vi "Verify position.vi"(8 "error in (no error)":errorcluster, 9 "Tolerance (um)":sgl=0.4, 10 "XYZ Position Input":T2={"Speed"=0, "Z Limit (um+/-)"=0.0, "Axes"="Z", "XYZ Coordinates"={"X"=0.0, "Y"=0.0, "Z"=0.0}} {"XYZ Coordinates"."Z" format="Z= %#_g"; "XYZ Coordinates"."Y" format="Y= %#_g"; "XYZ Coordinates"."X" format="X= %#_g"; "Z Limit (um+/-)" format="Z Limit = %.0f"; "Speed" format="Speed= %.0f"}, 11 "Scientifica XYZ Gen1 in":refnum<class "Scientifica XYZ Gen1.lvclass">) -> (0 "error out":errorcluster, 1 "XYZ Coordinates":T1 {"Z" format="Z= %#_g"; "Y" format="Y= %#_g"; "X" format="X= %#_g"}, 2 "Position reached":bool, 3 "Scientifica XYZ Gen1 out":refnum<class "Scientifica XYZ Gen1.lvclass">)   [LabVIEW 2020, in "TranslationStageClassStructure.lvlib" / "Scientifica XYZ Gen1.lvclass"]
uses:
  Scientifica XYZ Gen1.lvclass
  XYZ Stage Control/typedefs/XYZ_position_input.ctl
  XYZ Stage Control/typedefs/XYZ axes.ctl
  Typedefs/XYZ_coordinates.ctl
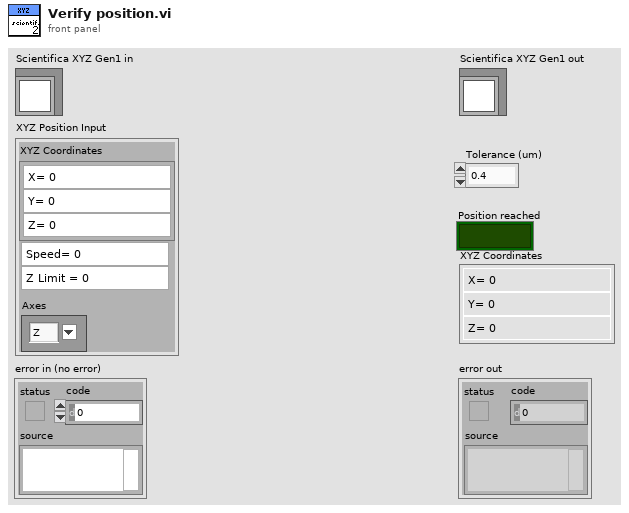
[diagram p1: front panel]
types:
  T1 = typedef "XYZ_coordinates.ctl" = cluster{"X":sgl, "Y":sgl, "Z":sgl}
  T2 = typedef "XYZ_position_input.ctl" = cluster{"Speed":i32, "Z Limit (um+/-)":sgl, "Axes":T3, "XYZ Coordinates":T1}
  T3 = typedef "XYZ axes.ctl" = string
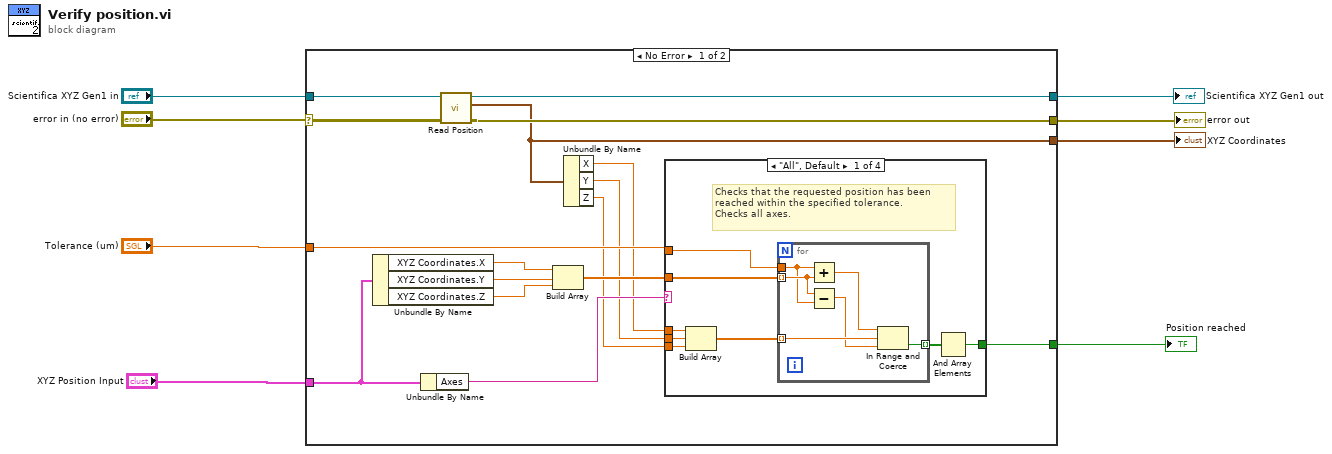
[diagram p0: block diagram]
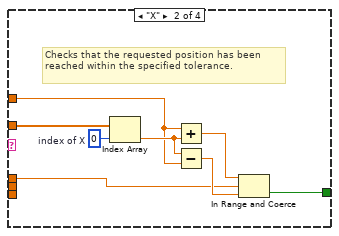
[diagram p2: hidden frame]
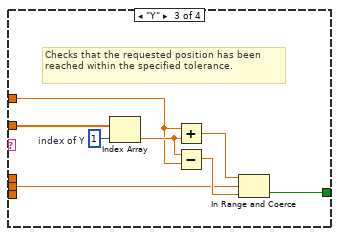
[diagram p3: hidden frame]
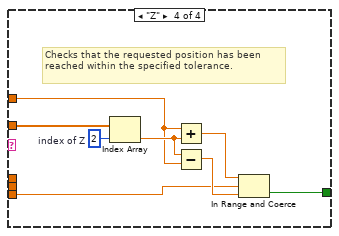
[diagram p4: hidden frame]
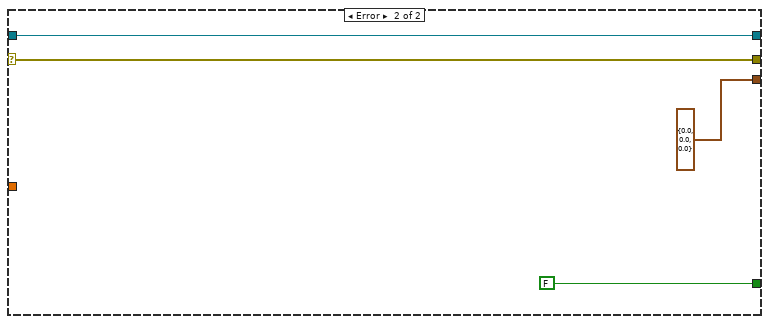
[diagram p5: hidden frame]
diagram:
  n1 = case shown="No Error" "error in (no error)" {
    selector: "error in (no error)" -> [w21 w65]
    tunnel: "Scientifica XYZ Gen1 in" -> [w24 w66]
    tunnel: "XYZ Position Input" -> [w23 _]
    tunnel: "Tolerance (um)" -> [w22 _]
    tunnel: [w20 w66] -> w4
    tunnel: [w19 w65] -> w3
    tunnel: [w18 FALSE] -> w2
    tunnel: [w9 T1 {"X"=0.0, "Y"=0.0, "Z"=0.0} ("XYZ Coordinates")] -> w1
    frame No Error {
      n2 = Unbundle By Name(w23) -> ("XYZ Coordinates.X"=w15:sgl, "XYZ Coordinates.Y"=w16:sgl, "XYZ Coordinates.Z"=w14:sgl)
      n3 = Unbundle By Name(w23) -> ("Axes"=w17:T3)
      n4 = call-dynamic "Read Position.vi"("error in (no error)"=w21, "Scientifica XYZ Gen1 in"=w24) -> ("error out"=w19:errorcluster, "XYZ Coordinates"=w9:T1, "Scientifica XYZ Gen1 out"=w20:refnum<class "Scientifica XYZ Gen1.lvclass">)  [unwired: 6 in, 1 out]
      n5 = Build Array(w15, w16, w14) -> (w13:sgl[])
      n6 = Unbundle By Name(w9) -> ("X"=w12:sgl, "Y"=w11:sgl, "Z"=w10:sgl)
      n7 = case shown="\"All\", Default" w17 {
        tunnel: w12 -> [w32 w40 _ _]
        tunnel: w11 -> [w31 _ w47 _]
        tunnel: w10 -> [w30 _ _ w55]
        tunnel: [w27 w39 w48 w56] -> w18
        tunnel: w13 -> [w26 w43 w51 w59]
        tunnel: w22 -> [w25 w41 w49 w57]
        frame "All", Default {
          # "Checks that the requested position has been reached within the specified tolerance.\nChecks all axes."
          n8 = Build Array(w32, w31, w30) -> (w29:sgl[])
          n9 = for {
            tunnel: w26 -> [w37] mode=indexing
            tunnel: w29 -> [w38] mode=indexing
            tunnel: [w34] -> w28 mode=indexing
            tunnel: w25 -> [w33]
            n10 = Add(x=w33, y=w37) -> (x+y=w36:sgl)
            n11 = Subtract(x=w37, y=w33) -> (x-y=w35:sgl)
            n12 = In Range and Coerce(upper limit=w36, x=w38, lower limit=w35) -> (In Range?=w34:bool)  [unwired: 1 out]
          }
          n13 = And Array Elements(Boolean array=w28) -> (logical AND=w27:bool)
        }
        frame "X" {
          w44 = 0  # index of X
          # "Checks that the requested position has been reached within the specified tolerance."
          n14 = Index Array(array=w43, index=w44) -> (element=w42:sgl)
          n15 = Add(x=w41, y=w42) -> (x+y=w46:sgl)
          n16 = Subtract(x=w42, y=w41) -> (x-y=w45:sgl)
          n17 = In Range and Coerce(upper limit=w46, x=w40, lower limit=w45) -> (In Range?=w39:bool)  [unwired: 1 out]
        }
        frame "Y" {
          w52 = 1  # index of Y
          # "Checks that the requested position has been reached within the specified tolerance."
          n18 = Index Array(array=w51, index=w52) -> (element=w50:sgl)
          n19 = Add(x=w49, y=w50) -> (x+y=w54:sgl)
          n20 = Subtract(x=w50, y=w49) -> (x-y=w53:sgl)
          n21 = In Range and Coerce(upper limit=w54, x=w47, lower limit=w53) -> (In Range?=w48:bool)  [unwired: 1 out]
        }
        frame "Z" {
          w60 = 2  # index of Z
          # "Checks that the requested position has been reached within the specified tolerance."
          n22 = Index Array(array=w59, index=w60) -> (element=w58:sgl)
          n23 = Add(x=w57, y=w58) -> (x+y=w62:sgl)
          n24 = Subtract(x=w58, y=w57) -> (x-y=w61:sgl)
          n25 = In Range and Coerce(upper limit=w62, x=w55, lower limit=w61) -> (In Range?=w56:bool)  [unwired: 1 out]
        }
      }
    }
    frame Error {
    }
  }
  "error out" <- w3
  "Scientifica XYZ Gen1 out" <- w4
  "Position reached" <- w2
  "XYZ Coordinates" <- w1
